vi "dpsk.vi"() -> ()   [LabVIEW 2014]
panel:
  out "decoded\n data 2":bool[](array[boolean])
  out "encoded data":bool[](array[boolean])
  in  "binary data":bool[](array[boolean])
  out "demodulated output":dynamicdata(graph)
  out "modulated DPSK":dynamicdata(graph)
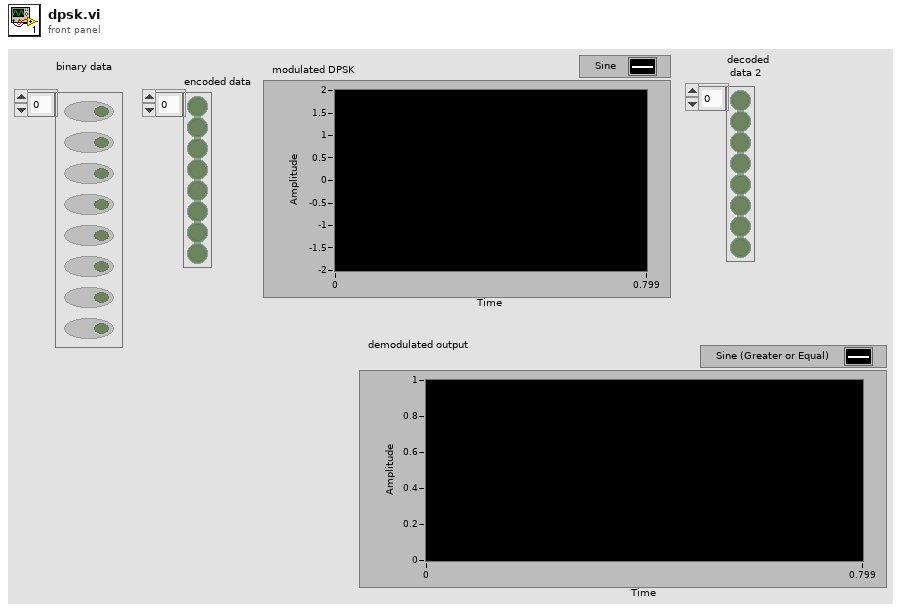
[diagram p1: front panel]
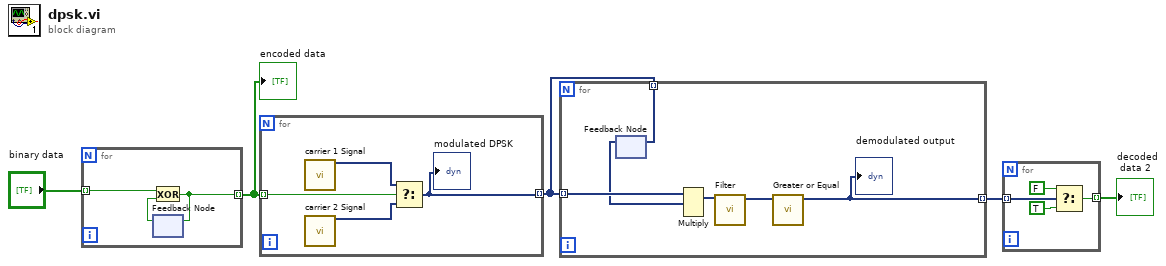
[diagram p0: block diagram]
diagram:
  n1 = for {
    tunnel: "binary data" -> [w8] mode=indexing
    tunnel: [w6] -> w4 mode=indexing
    n2 = feedback #1() -> (w7:bool)  [unwired: 1 in]
    n3 = Exclusive Or(1:w7, 2:w8) -> (0:w6:bool)
    n4 = feedback-in #1(w6) -> ()
  }
  "encoded data" <- w4
  n5 = for {
    tunnel: w4 -> [w10] mode=indexing
    tunnel: [w9] -> w1 mode=indexing
    n6 = call "carrier 1 Signal"() -> ("Sine"=w12:dynamicdata)  [unwired: 14 in, 1 out]
    n7 = call "carrier 2 Signal"() -> ("Sine"=w11:dynamicdata)  [unwired: 14 in, 1 out]
    n8 = Select(t=w12, s=w10, f=w11) -> (s? t:f=w9:dynamicdata)
    "modulated DPSK" <- w9
  }
  n9 = for {
    tunnel: w1 -> [w18] mode=indexing
    tunnel: [w16] -> w3 mode=indexing
    tunnel: w1 -> [w14] mode=indexing
    n10 = feedback #2() -> (w13:dynamicdata)  [unwired: 1 in]
    n11 = feedback-in #2(w14) -> ()
    n12 = Multiply(1:w13, 2:w18) -> (0:w17:dynamicdata)  [unwired: 1 in, 1 out]
    n13 = call "Filter"("Signal"=w17) -> ("Filtered Signal"=w15:dynamicdata)  [unwired: 9 in, 1 out]
    n14 = call "Greater or Equal"("Operand 1"=w15) -> ("Result"=w16:dynamicdata)  [unwired: 9 in, 1 out]
    "demodulated output" <- w16
  }
  n15 = for {
    tunnel: w3 -> [w20] mode=indexing
    tunnel: [w19] -> w2 mode=indexing
    n16 = Select(t=FALSE, s=w20, f=TRUE) -> (s? t:f=w19:bool)
  }
  "decoded\n data 2" <- w2
